vi "oa_Build DC Output Data (N Channels).vi"(0 "DC value out":dbl[][](array[numeric]), 1 "reset? (True)":bool=TRUE, 2 "X axis selection":u16(ring)=2 items=["Time", "Revolution", "RPM"], 5 "start points":dbl[](array[numeric]) format="%.2f", 7 "channel info":T1[](array[typedef]) {"pregain" format="%.2f"; "weighting filter" items=["Linear", "A-weighting", "B-weighting", "C-weighting", "ITU-R 468-4", "Dolby", "CCITT", "C-message", "Wb", "Wc", "Wd", "We", "Wf", "Wh", "Wj", "Wk", "Wm", "AES17 20 kHz lowpass", "AES17 40 kHz lowpass", "AES17 20 kHz highpass", "AES17 40 kHz highpass"]; "dB reference" format="%^.1e"; "engineering units" items=["custom..."=0, "V"=1, "A"=21, "C"=30, "pC"=31, "s"=32, "-"=29, "Pa"=2, "N"=20, "g"=3, "m/s^2"=4, "m/s"=5, "m"=6, "mm/s"=12, "mm"=13, "micron/s"=14, "micron"=15, "in/s^2"=7, "in/s"=8, "in"=9, "mil/s"=10, "mil"=11, "rad/s^2"=16, "rad/s"=17, "rad"=18, "deg/s^2"=26, "deg/s"=27, "deg"=28, "RPM"=22, "cycle/s^2"=23, "Hz"=24, "cycle"=25, "strain"=19]; "sensor sensitivity" format="%#_5f"}, 9 "samples/rev":dbl, 11 "error in (no error)":errorcluster, 12 "DC gap unit":u16(ring) items=["V", "EU"]) -> (4 "DC gaps":cluster{"X":dbl[], "Y":dbl[]}[](array[cluster]) {"Y" format="%.2f"; "X" format="%.2f"}, 8 "unit labels":cluster{"X unit":string, "gap unit":string}[](array[cluster]), 10 "pulse positions":dbl[](array[numeric]), 15 "error out":errorcluster)   [LabVIEW 2017, in "SoundVib_RefDataProcess.lvlib"]
uses:
  <vilib>/addons/Sound and Vibration/Order Analysis/Referece Data Processing/SoundVib_RefDataProcess.lvlib
  <vilib>/addons/_NISVFA/_Shared subVIs/Controls/svc_Channel Info.ctl
  <vilib>/addons/_NISVFA/_Shared subVIs/Controls/svc_Engineering Units Text Ring.ctl
  <vilib>/addons/_NISVFA/_Shared subVIs/Controls/svc_Weighting Filter Text Ring.ctl
  <vilib>/Analysis/1siggen.llb/Ramp Pattern by Samples.vi
  <vilib>/addons/Sound and Vibration/Order Analysis/Resample Order Tracking/SoundVib_Resampling.lvlib
  <vilib>/Analysis/NI_AALBase.lvlib
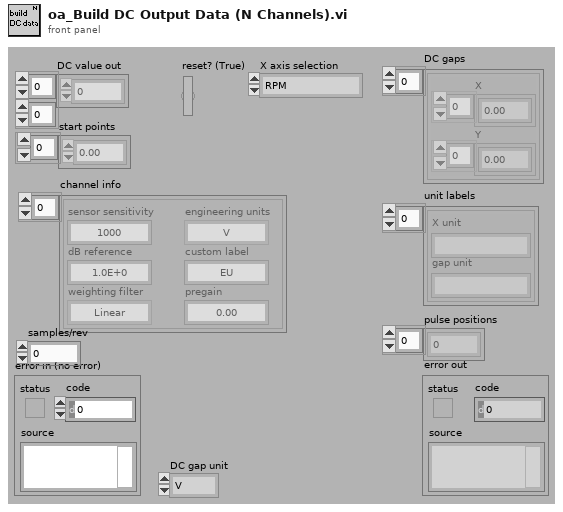
[diagram p1: front panel]
types:
  T1 = typedef "svc_Channel Info.ctl" = cluster{"sensor sensitivity":dbl, "engineering units":T2, "dB reference":dbl, "custom label":string, "weighting filter":T3, "pregain":dbl}
  T2 = typedef "svc_Engineering Units Text Ring.ctl" = u16
  T3 = typedef "svc_Weighting Filter Text Ring.ctl" = u16
  T4 = typedef "SoundVib_TachProcess.lvlib/speed profile.ctl" = cluster{"time [s]":dbl[], "speed [RPM]":dbl[]}
  T5 = cluster{"speed [RPM]":dbl[], "DC value out":dbl[]}
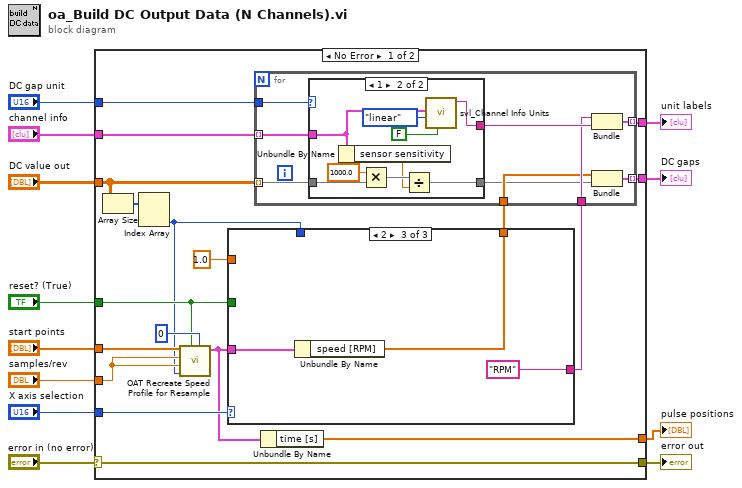
[diagram p0: block diagram]
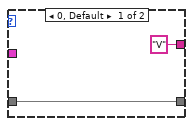
[diagram p2: hidden frame]
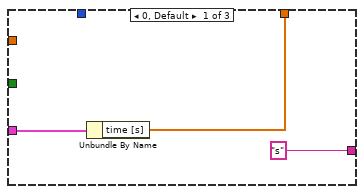
[diagram p3: hidden frame]
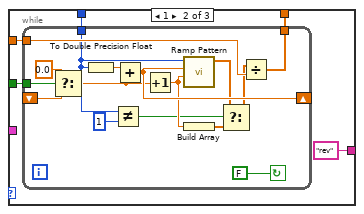
[diagram p4: hidden frame]
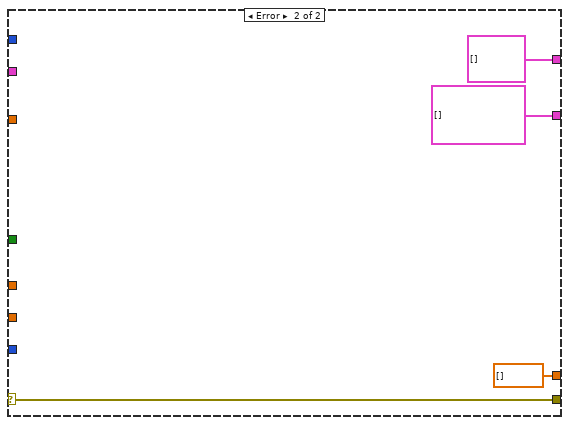
[diagram p5: hidden frame]
diagram:
  n1 = case shown="No Error" "error in (no error)" {
    selector: "error in (no error)" -> [w24 w81]
    tunnel: "X axis selection" -> [w28 _]
    tunnel: "reset? (True)" -> [w27 _]
    tunnel: [w26 cluster{dbl[], "DC value out":dbl[]}[] []] -> w10
    tunnel: "DC value out" -> [w22 _]
    tunnel: "start points" -> [w25 _]
    tunnel: [w24 w81] -> w6
    tunnel: [w19 cluster{string, "unit label":string}[] []] -> w4
    tunnel: "channel info" -> [w23 _]
    tunnel: "DC gap unit" -> [w17 _]
    tunnel: "samples/rev" -> [w16 _]
    tunnel: [w14 dbl[] [] ("time [s]")] -> w1
    frame No Error {
      n2 = Array Size(array=w22) -> (size(s)=w18:i32[])
      n3 = Index Array(array=w18) -> (element #2=w13:i32)  [unwired: 2 in, 1 out]
      n4 = call <vilib>:"OAT Recreate Speed Profile for Resample.vi"("lags"=0, "init/continue (init:T)"=w27, "output length"=w13, "decimation factor"=w16, "sample / rev"=w16, "time stamps in"=w25) -> ("speed profile"=w15:T4)  [unwired: 5 in]
      n5 = case shown="2" w28 {
        tunnel: w15 -> [w53 _ w77]
        tunnel: [w51 w58 w75] -> w21
        tunnel: 1.0 ("samples/rev") -> [_ w57 _]
        tunnel: w27 -> [_ w56 _]
        tunnel: ["s" "rev" "RPM"] -> w20
        tunnel: w13 -> [_ w54 _]
        frame 0, Default {
          n6 = Unbundle By Name(w53) -> ("time [s]"=w51:dbl[])
        }
        frame 1 {
          n7 = while {
            tunnel: [w74] -> w58
            tunnel: w57 -> [w73]
            tunnel: w56 -> [w71]
            shift-right: [w70] -> _
            shift-left: _ -> [w59]
            tunnel: w54 -> [w69]
            stop <- FALSE continue-if-true
            n8 = Select(t=0.0 ("f"), s=w71, f=w59) -> (s? t:f=w67:dbl)
            n9 = To Double Precision Float(number=w69) -> (double precision float=w60:dbl)
            n10 = Not Equal?(x=w69, y=1) -> (x != y?=w64:bool)
            n11 = Add(x=w60, y=w67) -> (x+y=w70:dbl)
            n12 = Increment(x=w67) -> (x+1=w65:dbl)
            n13 = call-poly <vilib>:"Ramp Pattern.vi"("start"=w65, "end"=w70, "samples"=w69) -> ("Ramp Pattern"=w63:dbl[])  [unwired: 7 in, 1 out]
            n14 = Build Array(w65) -> (w62:dbl[])
            n15 = Select(t=w63, s=w64, f=w62) -> (s? t:f=w61:dbl[])
            n16 = Divide(x=w61, y=w73) -> (x/y=w74:dbl[])
          }
        }
        frame 2 {
          n17 = Unbundle By Name(w77) -> ("speed [RPM]"=w75:dbl[])
        }
      }
      n18 = for {
        tunnel: [w39] -> w26 mode=indexing
        tunnel: w22 -> [w32] mode=indexing
        tunnel: w23 -> [w38] mode=indexing
        tunnel: w21 -> [w34]
        tunnel: w20 -> [w36]
        tunnel: [w35] -> w19 mode=indexing
        tunnel: w17 -> [w33]
        n19 = case shown="1" w33 {
          tunnel: w38 -> [_ w44]
          tunnel: ["V" ("unit label") w48] -> w37
          tunnel: w32 -> [w41 w47]
          tunnel: [w41 w42] -> w31
          frame 0, Default {
          }
          frame 1 {
            n20 = Unbundle By Name(w44) -> ("sensor sensitivity"=w43:dbl)
            n21 = Multiply(x=1000.0, y=w47) -> (x*y=w45:dbl[])
            n22 = Divide(x=w45, y=w43) -> (x/y=w42:dbl[])
            n23 = call <vilib>:"svl_Channel Info Units.vi"("include weighting if dB On FALSE"=FALSE, "linear/dB"=enum16{"linear", "dB"}."linear", "channel info"=w44) -> ("unit label"=w48:string)  [unwired: 7 in, 1 out]
          }
        }
        n24 = Bundle(w36, "unit label"=w37) -> (w35:cluster{string, "unit label":string})  [unwired: 1 in]
        n25 = Bundle("speed [RPM]"=w34, "DC value out"=w31) -> (w39:T5)  [unwired: 1 in]
      }
      n26 = Unbundle By Name(w15) -> ("time [s]"=w14:dbl[])
    }
    frame Error {
    }
  }
  "error out" <- w6
  "DC gaps" <- w10
  "unit labels" <- w4
  "pulse positions" <- w1
